vi "sub vi - GET ALL TEMP v7.vi"(0 "LA01-EN":bool, 1 "simulate":bool, 5 "LA02-EN":bool, 7 "LA03-EN":bool, 9 "LA04-EN":bool, 11 "LA05-EN":bool, 12 "Gen Cal Value":dbl) -> (2 "LOOP TIME":dbl, 3 "ID":T1, 4 "LA01 TEMP":T2, 6 "LA02 TEMP":T2, 8 "LA03 TEMP":T2, 10 "LA04 TEMP":T2, 13 "Zero Counters":u64[](array[numeric]), 14 "error":bool, 15 "LA05 TEMP":T2)   [LabVIEW 2017]
uses:
  program files/Global display 4.vi
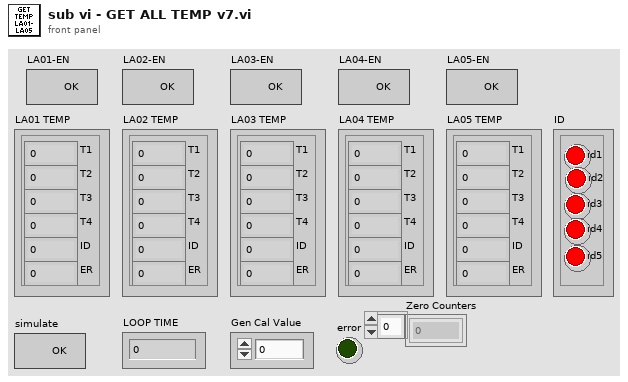
[diagram p1: front panel]
types:
  T1 = cluster{"id1":bool, "id2":bool, "id3":bool, "id4":bool, "id5":bool}
  T2 = cluster{"T1":dbl, "T2":dbl, "T3":dbl, "T4":dbl, "ID":dbl, "ER":dbl}
  T3 = cluster{"1 TL":dbl, "1 TN":dbl, "2 TL":dbl, "2 TN":dbl, "ID":dbl, "ER":dbl}
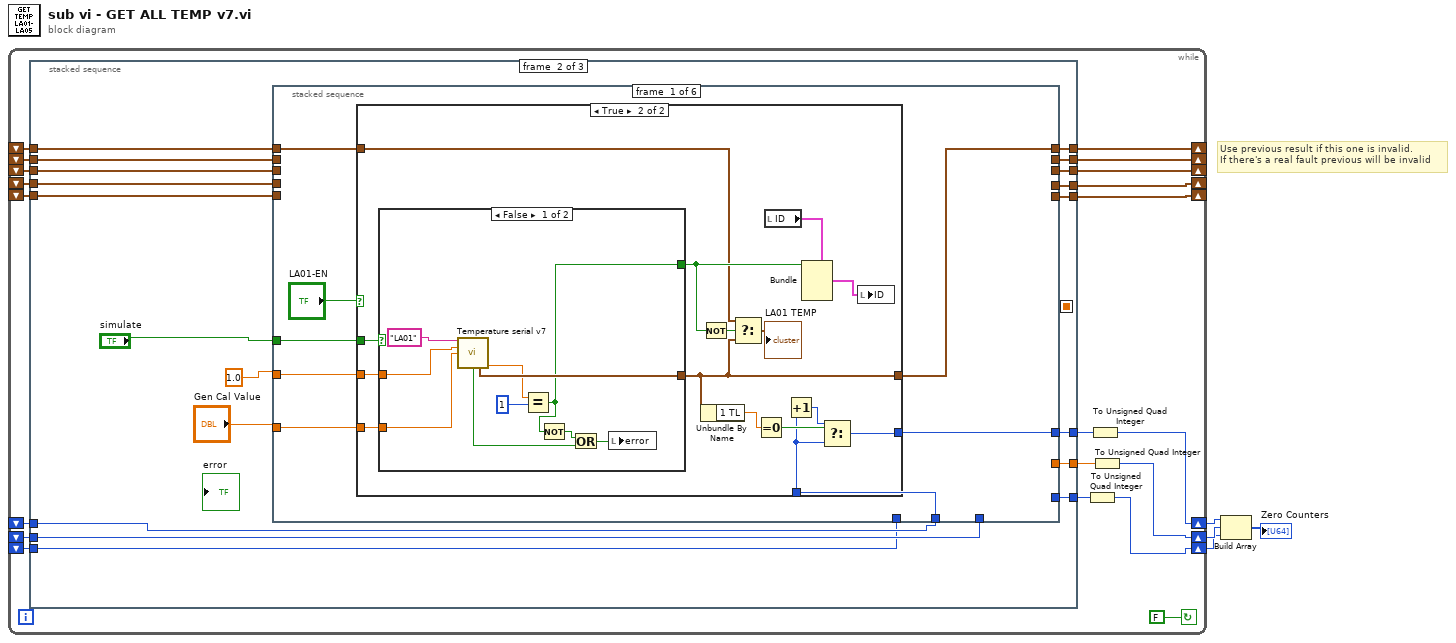
[diagram p0: block diagram]
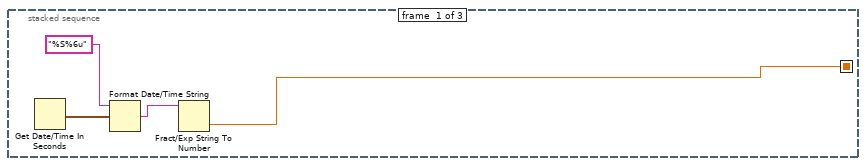
[diagram p2: hidden frame]
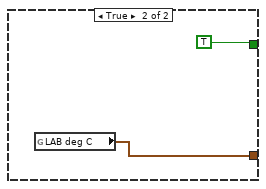
[diagram p4: hidden frame]
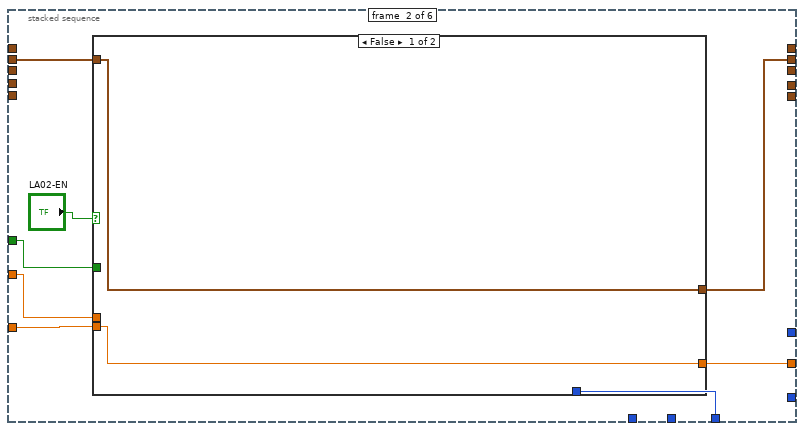
[diagram p5: hidden frame]
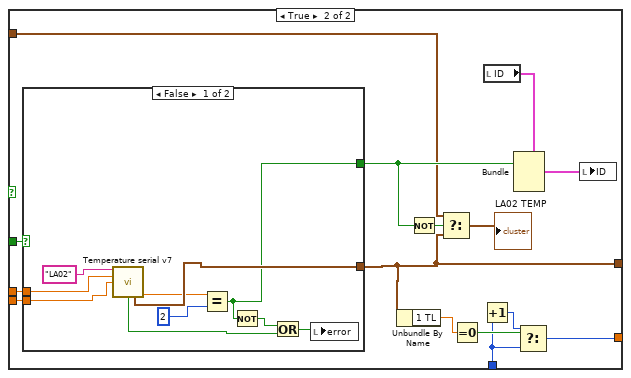
[diagram p6: hidden frame]
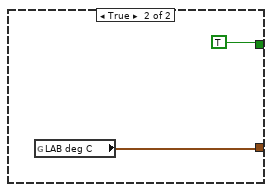
[diagram p7: hidden frame]
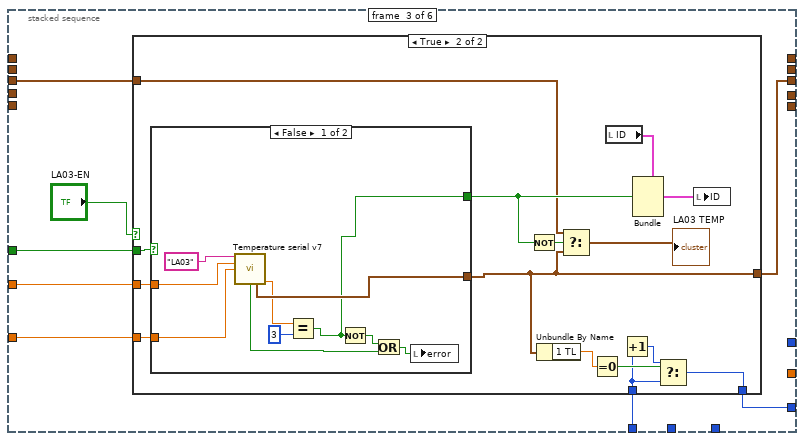
[diagram p8: hidden frame]
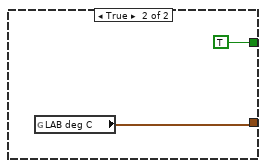
[diagram p10: hidden frame]
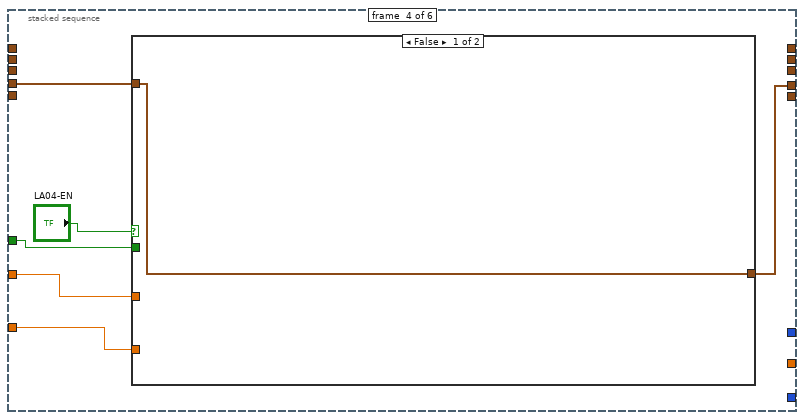
[diagram p11: hidden frame]
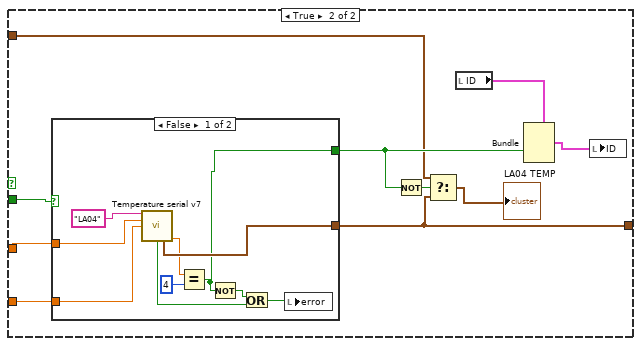
[diagram p12: hidden frame]
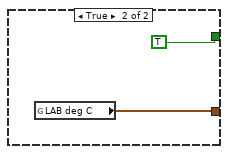
[diagram p13: hidden frame]
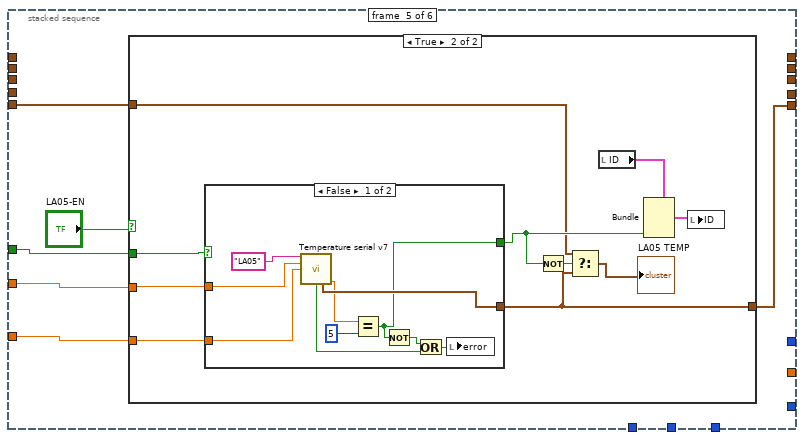
[diagram p14: hidden frame]
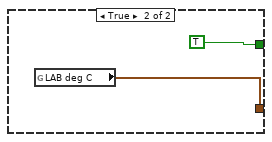
[diagram p16: hidden frame]
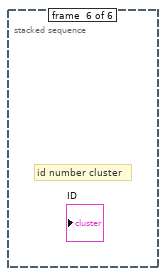
[diagram p17: hidden frame]
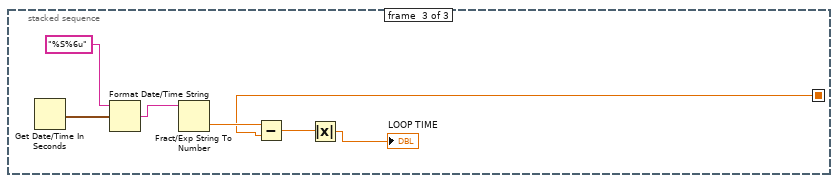
[diagram p18: hidden frame]
diagram:
  # "Use previous result if this one is invalid.\nIf there's a real fault previous will be invalid"
  n1 = while {
    shift-right: [w17] -> w4
    shift-left: _ -> [w23]
    shift-right: [w16] -> w3
    shift-left: _ -> [w21]
    shift-right: [w15] -> w2
    shift-left: _ -> [w18]
    shift-right: [w13] -> _
    shift-left: _ -> [w14]
    shift-right: [w11] -> _
    shift-left: _ -> [w12]
    shift-right: [w9] -> _
    shift-left: _ -> [w10]
    shift-right: [w8] -> _
    shift-left: _ -> [w7]
    shift-right: [w6] -> _
    shift-left: _ -> [w5]
    stop <- FALSE continue-if-true
    n2 = stacked-sequence {
      seq-local: [w25 _ _] -> [_ _ w219]
      tunnel: w23 -> [_ w44 _]
      tunnel: [_ w43 _] -> w22
      tunnel: w21 -> [_ w42 _]
      tunnel: [_ w41 _] -> w20
      tunnel: [_ w40 _] -> w19
      tunnel: w18 -> [_ w39 _]
      tunnel: w14 -> [_ w38 _]
      tunnel: [_ w37 _] -> w13
      tunnel: w12 -> [_ w36 _]
      tunnel: [_ w35 _] -> w11
      tunnel: w10 -> [_ w34 _]
      tunnel: [_ w33 _] -> w9
      tunnel: [_ w32 _] -> w8
      tunnel: w7 -> [_ w31 _]
      tunnel: [_ w30 _] -> w6
      tunnel: w5 -> [_ w29 _]
      frame #0 {
        n3 = Get Date/Time In Seconds() -> (seconds since 1Jan1904=w28:timestamp)
        n4 = Format Date/Time String(time format string (%c)="%S%6u", seconds (now)=w28) -> (date/time string=w26:string)  [unwired: 1 in]
        n5 = Fract/Exp String To Number(string=w26) -> (number=w25:dbl)  [unwired: 3 in, 1 out]
      }
      frame #1 {
        n6 = stacked-sequence {
          tunnel: sgl 1.0 -> [w55 w92 w129 w164 w193 _]
          tunnel: "Gen Cal Value" -> [w54 w91 w128 w163 w192 _]
          tunnel: "simulate" -> [w52 w89 w126 w161 w190 _]
          tunnel: w44 -> [w51 _ _ _ _ _]
          tunnel: [w50 _ _ _ _ _] -> w43
          tunnel: w42 -> [_ w88 _ _ _ _]
          tunnel: [_ w87 _ _ _ _] -> w41
          tunnel: [_ _ w125 _ _ _] -> w40
          tunnel: w39 -> [_ _ w124 _ _ _]
          tunnel: w38 -> [w49 _ _ _ _ _]
          tunnel: [w48 _ _ _ _ _] -> w37
          tunnel: w36 -> [_ w86 _ _ _ _]
          tunnel: [_ w85 _ _ _ _] -> w35
          tunnel: w34 -> [_ _ w123 _ _ _]
          tunnel: [_ _ w122 _ _ _] -> w33
          tunnel: [_ _ _ w160 _ _] -> w32
          tunnel: w31 -> [_ _ _ w159 _ _]
          tunnel: [_ _ _ _ w189 _] -> w30
          tunnel: w29 -> [_ _ _ _ w188 _]
          frame #0 {
            n7 = case shown="True" "LA01-EN" {
              tunnel: w55 -> [_ w72]
              tunnel: w54 -> [_ w71]
              tunnel: w52 -> [_ w70]
              tunnel: w51 -> [w57 w63]
              tunnel: [w57 w64] -> w50
              tunnel: w49 -> [w56 w60]
              tunnel: [w56 w58] -> w48
              frame False {
              }
              frame True {
                n8 = case shown="False" w70 {
                  tunnel: w72 -> [w81 _]
                  tunnel: w71 -> [w80 _]
                  tunnel: [w79 w84] -> w58
                  tunnel: [w73 TRUE] -> w62
                  frame False {
                    n9 = call "Temperature serial v7.vi"("Command String"="LA01", "Time Out (S)"=w81, "CALIB"=w80) -> ("error"=w76:bool, "output cluster"=w79:cluster{dbl, dbl, dbl, dbl, i32, "error #":dbl}, "Unit ID"=w75:dbl)  [unwired: 6 in, 4 out]
                    n10 = Equal?(x=w75, y=1) -> (x = y?=w73:bool)
                    n11 = Not(x=w73) -> (.not. x?=w74:bool)
                    n12 = Or(x=w74, y=w76) -> (x .or. y?=w77:bool)
                    n13 = local write "error"(w77) -> ()
                  }
                  frame True {
                    n14 = global read "Global display 4.vi" "LAB deg C"() -> (w84:T3)
                  }
                }
                n15 = Not(x=w62) -> (.not. x?=w61:bool)
                n16 = Unbundle By Name(w58) -> ("1 TL"=w67:dbl)
                n17 = Select(t=w60, s=w61, f=w58) -> (s? t:f=→"LA01 TEMP":T3)
                n18 = Equal To 0?(x=w67) -> (x = 0?=w66:bool)
                n19 = local read "ID"() -> (w69:T1)
                n20 = Increment(x=w63) -> (x+1=w65:u64)
                n21 = Bundle(cluster=w69, "id1"=w62) -> (w68:T1)  [unwired: 4 in]
                n22 = Select(t=w65, s=w66, f=w63) -> (s? t:f=w64:u64)
                n23 = local write "ID"(w68) -> ()
              }
            }
          }
          frame #1 {
            n24 = case shown="False" "LA02-EN" {
              tunnel: w92 -> [_ w109]
              tunnel: w91 -> [w94 w108]
              tunnel: w89 -> [_ w107]
              tunnel: w88 -> [_ w101]
              tunnel: [w94 w100] -> w87
              tunnel: w86 -> [w93 w97]
              tunnel: [w93 w95] -> w85
              frame False {
              }
              frame True {
                n25 = case shown="False" w107 {
                  tunnel: w109 -> [w118 _]
                  tunnel: w108 -> [w117 _]
                  tunnel: [w116 w121] -> w95
                  tunnel: [w110 TRUE] -> w98
                  frame False {
                    n26 = call "Temperature serial v7.vi"("Command String"="LA02", "Time Out (S)"=w118, "CALIB"=w117) -> ("error"=w114:bool, "output cluster"=w116:cluster{dbl, dbl, dbl, dbl, i32, "error #":dbl}, "Unit ID"=w112:dbl)  [unwired: 6 in, 4 out]
                    n27 = Equal?(x=w112, y=2) -> (x = y?=w110:bool)
                    n28 = Not(x=w110) -> (.not. x?=w111:bool)
                    n29 = Or(x=w111, y=w114) -> (x .or. y?=w115:bool)
                    n30 = local write "error"(w115) -> ()
                  }
                  frame True {
                    n31 = global read "Global display 4.vi" "LAB deg C"() -> (w121:T3)
                  }
                }
                n32 = Unbundle By Name(w95) -> ("1 TL"=w104:dbl)
                n33 = Not(x=w98) -> (.not. x?=w99:bool)
                n34 = Select(t=w97, s=w99, f=w95) -> (s? t:f=→"LA02 TEMP":T3)
                n35 = Equal To 0?(x=w104) -> (x = 0?=w103:bool)
                n36 = Increment(x=w101) -> (x+1=w102:u64)
                n37 = local read "ID"() -> (w106:T1)
                n38 = Bundle(cluster=w106, "id2"=w98) -> (w105:T1)  [unwired: 4 in]
                n39 = Select(t=w102, s=w103, f=w101) -> (s? t:f=w100:u64)
                n40 = local write "ID"(w105) -> ()
              }
            }
          }
          frame #2 {
            n41 = case shown="True" "LA03-EN" {
              tunnel: w129 -> [_ w146]
              tunnel: w128 -> [_ w145]
              tunnel: w126 -> [_ w144]
              tunnel: [w131 w138] -> w125
              tunnel: w124 -> [w131 w137]
              tunnel: w123 -> [w130 w134]
              tunnel: [w130 w132] -> w122
              frame False {
              }
              frame True {
                n42 = case shown="False" w144 {
                  tunnel: w146 -> [w155 _]
                  tunnel: w145 -> [w154 _]
                  tunnel: [w153 w158] -> w132
                  tunnel: [w147 TRUE] -> w135
                  frame False {
                    n43 = call "Temperature serial v7.vi"("Command String"="LA03", "Time Out (S)"=w155, "CALIB"=w154) -> ("error"=w150:bool, "output cluster"=w153:cluster{dbl, dbl, dbl, dbl, i32, "error #":dbl}, "Unit ID"=w149:dbl)  [unwired: 6 in, 4 out]
                    n44 = Equal?(x=w149, y=3) -> (x = y?=w147:bool)
                    n45 = Not(x=w147) -> (.not. x?=w148:bool)
                    n46 = Or(x=w148, y=w150) -> (x .or. y?=w152:bool)
                    n47 = local write "error"(w152) -> ()
                  }
                  frame True {
                    n48 = global read "Global display 4.vi" "LAB deg C"() -> (w158:T3)
                  }
                }
                n49 = Not(x=w135) -> (.not. x?=w136:bool)
                n50 = Unbundle By Name(w132) -> ("1 TL"=w141:dbl)
                n51 = Select(t=w134, s=w136, f=w132) -> (s? t:f=→"LA03 TEMP":T3)
                n52 = Equal To 0?(x=w141) -> (x = 0?=w140:bool)
                n53 = local read "ID"() -> (w143:T1)
                n54 = Increment(x=w137) -> (x+1=w139:u64)
                n55 = Bundle(cluster=w143, "id3"=w135) -> (w142:T1)  [unwired: 4 in]
                n56 = Select(t=w139, s=w140, f=w137) -> (s? t:f=w138:u64)
                n57 = local write "ID"(w142) -> ()
              }
            }
          }
          frame #3 {
            n58 = case shown="False" "LA04-EN" {
              tunnel: w164 -> [_ w175]
              tunnel: w163 -> [_ w174]
              tunnel: w161 -> [_ w173]
              tunnel: [w165 w168] -> w160
              tunnel: w159 -> [w165 w166]
              frame False {
              }
              frame True {
                n59 = case shown="False" w173 {
                  tunnel: w175 -> [w184 _]
                  tunnel: w174 -> [w183 _]
                  tunnel: [w182 w187] -> w168
                  tunnel: [w176 TRUE] -> w169
                  frame False {
                    n60 = call "Temperature serial v7.vi"("Command String"="LA04", "Time Out (S)"=w184, "CALIB"=w183) -> ("error"=w180:bool, "output cluster"=w182:cluster{dbl, dbl, dbl, dbl, i32, "error #":dbl}, "Unit ID"=w178:dbl)  [unwired: 6 in, 4 out]
                    n61 = Equal?(x=w178, y=4) -> (x = y?=w176:bool)
                    n62 = Not(x=w176) -> (.not. x?=w177:bool)
                    n63 = Or(x=w177, y=w180) -> (x .or. y?=w181:bool)
                    n64 = local write "error"(w181) -> ()
                  }
                  frame True {
                    n65 = global read "Global display 4.vi" "LAB deg C"() -> (w187:T3)
                  }
                }
                n66 = Not(x=w169) -> (.not. x?=w170:bool)
                n67 = Select(t=w166, s=w170, f=w168) -> (s? t:f=→"LA04 TEMP":T3)
                n68 = local read "ID"() -> (w172:T1)
                n69 = Bundle(cluster=w172, "id4"=w169) -> (w171:T1)  [unwired: 4 in]
                n70 = local write "ID"(w171) -> ()
              }
            }
          }
          frame #4 {
            n71 = case shown="True" "LA05-EN" {
              tunnel: w193 -> [_ w204]
              tunnel: w192 -> [_ w203]
              tunnel: w190 -> [_ w202]
              tunnel: [w194 w196] -> w189
              tunnel: w188 -> [w194 w197]
              frame False {
              }
              frame True {
                n72 = case shown="False" w202 {
                  tunnel: w204 -> [w213 _]
                  tunnel: w203 -> [w212 _]
                  tunnel: [w211 w216] -> w196
                  tunnel: [w205 TRUE] -> w198
                  frame False {
                    n73 = call "Temperature serial v7.vi"("Command String"="LA05", "Time Out (S)"=w213, "CALIB"=w212) -> ("error"=w209:bool, "output cluster"=w211:cluster{dbl, dbl, dbl, dbl, i32, "error #":dbl}, "Unit ID"=w207:dbl)  [unwired: 6 in, 4 out]
                    n74 = Equal?(x=w207, y=5) -> (x = y?=w205:bool)
                    n75 = Not(x=w205) -> (.not. x?=w206:bool)
                    n76 = Or(x=w206, y=w209) -> (x .or. y?=w210:bool)
                    n77 = local write "error"(w210) -> ()
                  }
                  frame True {
                    n78 = global read "Global display 4.vi" "LAB deg C"() -> (w216:T3)
                  }
                }
                n79 = Not(x=w198) -> (.not. x?=w199:bool)
                n80 = Select(t=w197, s=w199, f=w196) -> (s? t:f=→"LA05 TEMP":T3)
                n81 = local read "ID"() -> (w201:T1)
                n82 = Bundle(cluster=w201, "id5"=w198) -> (w200:T1)  [unwired: 4 in]
                n83 = local write "ID"(w200) -> ()
              }
            }
          }
          frame #5 {
            # "id number cluster"
          }
        }
      }
      frame #2 {
        n84 = Get Date/Time In Seconds() -> (seconds since 1Jan1904=w223:timestamp)
        n85 = Format Date/Time String(time format string (%c)="%S%6u", seconds (now)=w223) -> (date/time string=w221:string)  [unwired: 1 in]
        n86 = Fract/Exp String To Number(string=w221) -> (number=w220:dbl)  [unwired: 3 in, 1 out]
        n87 = Subtract(x=w220, y=w219) -> (x-y=w218:dbl)
        n88 = Absolute Value(x=w218) -> (abs(x)=→"LOOP TIME":dbl)
      }
    }
    n89 = To Unsigned Quad Integer(1:w19) -> (0:w15:u64)
    n90 = To Unsigned Quad Integer(1:w22) -> (0:w17:u64)
    n91 = To Unsigned Quad Integer(1:w20) -> (0:w16:u64)
  }
  n92 = Build Array(w4, w3, w2) -> (→"Zero Counters":u64[])
